vi "SemErrorLog.vi"() -> ()   [LabVIEW 2019]
panel:
  out "SemErrorLog":T1
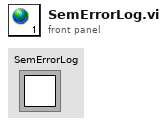
[diagram p1: front panel]
types:
  T1 = typedef "Semaphore RefNum" = refnum<k1>
diagram:
